vi "Do Non-Critical Stuff.vi"() -> ()   [LabVIEW 2017]
panel:
  out "Torque Chart":dbl(graph)
  out "Uncertainty Contributions":dbl[](array[numeric])
  out "Discharge Pressure Random Uncertainty":dbl
  out "Suction Pressure Random Uncertainty":dbl
  out "Suction Temperature Random Uncertainty":dbl
  out "size(s)":i32
  out "varclusterarray":T1(array[cluster])
  in  "units":enum16{"SI", "IP"}(ring)
  out "Hevap,inlet":string
  out "Psat(130F)":string
  out "Density":string
  out "Psat(45F)":string
  out "x > y?":bool
  out "x .and. y?":bool
  out "queue out":refnum<queue>
  out "DT Subcool":dbl
  out "DT Superheat":dbl
  out "Volumetric Efficiency":dbl
  out "Capacity":dbl
  out "Isentropic Efficiency":dbl
  in  "Tab Control":enum32{"Test Information", "Test Data"}(tab)
  in  "Test Matrix File":path=path "C:/Users/betsrgadmin/Desktop/80_Labview/80_Ton_Labview/test_matrix_labview_40ton_1234ze.csv"
  in  "Systematic Uncertainty of Pdis":dbl=0.375
  in  "Systematic Uncertainty of Psuc":dbl=0.1
  in  "Systematic Uncertainty of Tsuc":dbl=0.2
  in  "Build Sheet Directory":path=path "C:/Users/betsrgadmin/Desktop/80_Labview/80_Ton_Labview/Build_Sheets"
  in  "Data Root Directory":path=path "C:/Users/betsrgadmin/Desktop/80_Labview/80_Ton_Labview/Test_Data"
  in  "Debug?":bool
  in  "Fluid":u16(ring)=220 items=["AIR.MIX", "AMARILLO.MIX", "EKOFISK.MIX", "GLFCOAST.MIX", "HIGHCO2.MIX", "HIGHN2.MIX", "NGSAMPLE.MIX", "R401A.MIX", "R401B.MIX", "R401C.MIX", "R402A.MIX", "R402B.MIX", "R403A.MIX", "R403B.MIX", "R405A.MIX", "R406A.MIX", "R407A.MIX", "R407B.MIX", "R407C.MIX", "R407D.MIX", "R407E.MIX", "R408A.MIX", "R409A.MIX", "R409B.MIX", "R410A.PPF", "R410B.MIX", "R411A.MIX", "R411B.MIX", "R412A.MIX", "R413A.MIX", "R414B.MIX", "R415A.MIX", "R415B.MIX", "R416A.MIX", "R417A.MIX", "R417B.MIX", "R417C.MIX", "R418A.MIX", "R419A.MIX", "R419B.MIX", "R420A.MIX", "R421A.MIX", "R421B.MIX", "R422A.MIX", "R422B.MIX", "R422C.MIX", "R422D.MIX", "R423A.MIX", "R424A.MIX", "R425A.MIX", "R426A.MIX", "R427A.MIX", "R428A.MIX", "R429A.MIX", "R430A.MIX", "R431A.MIX", "R432A.MIX", "R433A.MIX", "R433B.MIX", "R433C.MIX", "R434A.MIX", "R435A.MIX", "R436A.MIX", "R436B.MIX", "R437A.MIX", "R438A.MIX", "R439A.MIX", "R440A.MIX", "R441A.MIX", "R442A.MIX", "R443A.MIX", "R444A.MIX", "R444B.MIX", "R445A.MIX", "R446A.MIX", "R447A.MIX", "R448A.MIX", "R449A.MIX", "R449B.MIX", "R450A.MIX", "R451A.MIX", "R451B.MIX", "R452A.MIX", "R452B.MIX", "R452C.MIX", "R453A.MIX", "R454A.MIX", "R454B.MIX", "R454C.MIX", "R455A.MIX", "R456A.MIX", "R457A.MIX", "R459A.MIX", "R459B.MIX", "R460A.MIX", "R460B.MIX", "R500.MIX", "R501.MIX", "R502.MIX", "R503.MIX", "R504.MIX", "R507A.MIX", "R508A.MIX", "R508B.MIX", "R509A.MIX", "R510A.MIX", "R511A.MIX", "R512A.MIX", "R513A.MIX", "R513B.MIX", "R515A.MIX", "ammonia.fld", "butane.fld", "ethane.fld", "propane.fld", "R11.fld", "R113.fld", "R114.fld", "R115.fld", "R116.fld", "R12.fld", "R123.fld", "R124.fld", "R125.fld", "R13.fld", "R134a.fld", "R14.fld", "R141b.fld", "R142b.fld", "R143a.fld", "R152a.fld", "R161.fld", "R21.fld", "R218.fld", "R22.fld", "R227ea.fld", "R23.fld", "R236ea.fld", "R236fa.fld", "R245ca.fld", "R245fa.fld", "R32.fld", "R41.fld", "R1216.fld", "RC318.fld", "water.fld", "1butene.fld", "acetone.fld", "argon.fld", "benzene.fld", "c1cc6.fld", "c2butene.fld", "c3cc6.fld", "c4f10.fld", "c5f12.fld", "c11.fld", "c12.fld", "cf3i.fld", "CO.fld", "CO2.fld", "COS.fld", "cyclohex.fld", "cyclopen.fld", "cyclopro.fld", "D2.fld", "D2O.fld", "D4.fld", "D5.fld", "D6.fld", "decane.fld", "dee.fld", "dmc.fld", "dme.fld", "ebenzene.fld", "ethanol.fld", "ethylene.fld", "flourine.fld", "H2S.fld", "HCl.fld", "helium.fld", "heptane.fld", "hexane.fld", "hydrogen.fld", "ibutene.fld", "ihexane.fld", "ioctane.fld", "ipentane.fld", "isobutan.fld", "krypton.fld", "MD2M.fld", "MD3M.fld", "MD4M.fld", "MDM.fld", "methane.fld", "methanol.fld", "mlinolea.fld", "mlinolen.fld", "MM.fld", "moleate.fld", "mpalmita.fld", "mstearat.fld", "mxylene.fld", "N2O.fld", "neon.fld", "neopentn.fld", "NF3.fld", "nitrogen.fld", "nonane.fld", "novec649.fld", "octane.fld", "orthohyd.fld", "oxygen.fld", "parahyd.fld", "pentane.fld", "propylen.fld", "propyne.fld", "pxylene.fld", "R365MFC.fld", "R1233zd.fld", "R1234yf.fld", "R1234ze.fld", "RE143a.fld", "RE245cb2.fld", "RE245fa2.fld", "RE347mcc.fld", "sf6.fld", "SO2.fld", "T2butene.fld", "xenon.fld"]
  out "Number in Queue":i32
  in  "Save Data":bool
  in  "Override Build\nFile Write":bool=TRUE
  in  "Purpose of Test (NO COMMAS)":string
  in  "Tester":string(combo)="J Singleton"
  in  "Test Comments (NO COMMAS)":string
  in  "Build Number":string="40TonSpool_ze"
  in  "Test Request\n    Number":string="1"
  out "Raw Data Directory Path":path
  out "Raw Data File Path":path
  in  "Points to Aquire":i32=1000
  in  "Compressor Displacement Volume (m^3)":dbl=0.002143428
  in  "Nominal Rotational Speed Hz":dbl=60.0
  out "Nominal Capacity kW":dbl
  in  "Units":string(combo)="IP"
  in  "# Motor Poles":dbl=4.0
  in  "Dump Queue":bool
  in  "Test Number in Matrix you want\n(Use this if manually changing to new setpoint. Otherwise, SP will change automatically when saved.)":i32=1
  out "Number in matrix being tested":i32
  out "Total Suction Temperature Uncertainty":dbl
  out "Total Suction Pressure Uncertainty":dbl
  out "Total Discharge Pressure Uncertainty":dbl
  out "Psuc Random Contribution to Total":dbl
  out "Tsuc Random Contribution to Total":dbl
  out "Pdis Random Contribution to Total":dbl
  in  "Collect Transient":bool
  in  "percentage of random uncertainty allowed":dbl=10.0 format="%#_13g"
  in  "Economizer used?":bool
  out "?":cluster{dbl, string, string}[](array[cluster])
  out "?":cluster{dbl, string, string}[](array[cluster])
  in  "?":T2(tab)
  in  "?":T3(tab)
  out "Primary Pressure Plot":dbl[][](graph)
  out "Secondary Pressure Plot":dbl[][](graph)
  out "Primary Pressure Plot 2":dbl[][](graph)
  in  "?":T4(tab)
  out "Primary Temperature Plot":dbl[][](graph)
  out "Secondary Temperature Plot":dbl[][](graph)
  out "Primary Temperature Plot 2":dbl[][](graph)
  out "Oil Mass Flow Plot":dbl[][](graph)
  out "Mass Flow Plot":dbl[][](graph)
  out "DTsup/DTsub Plot":dbl[][](graph)
  out "Efficiency Plot":dbl[][](graph)
  out "?":dbl[][](graph)
  out "Random uncertainties":dbl[][](graph)
  out "?":cluster{dbl, string, string}[](array[cluster]) {"?" format="%#_5g"}
  out "?":cluster{dbl, string, string}[](array[cluster]) {"?" format="%#_3g"}
  out "?":cluster{dbl, string, string}[](array[cluster]) {"?" format="%#_3g"}
  out "?":cluster{dbl, string, string}[](array[cluster]) {"?" format="%#_4g"}
  in  "stop":bool
  out "?":cluster{dbl, string, string}[](array[cluster])
  out "?":cluster{dbl, string, string}[](array[cluster])
  # "Seth was present here."
  # "Test Information"
  # "Compressor Information"
  # "Data Collection Information"
  # "Code will automatically save the test \ncondtion when the uncertainty is \nminimized. The condition can be saved \nmanually by pressing \"Save Data\""
  # "The code will not begin queuing data until the pressures\nare within +/- 1% and the temperature is within +/-\n1 F of the setpoint (ASHRAE  2010 compressor testing \nstandard). If a different threshold is desired, or a \ntransient condition is being tested, press \"Collect Transient\" to begin queuing data."
  # "Measurement Plots"
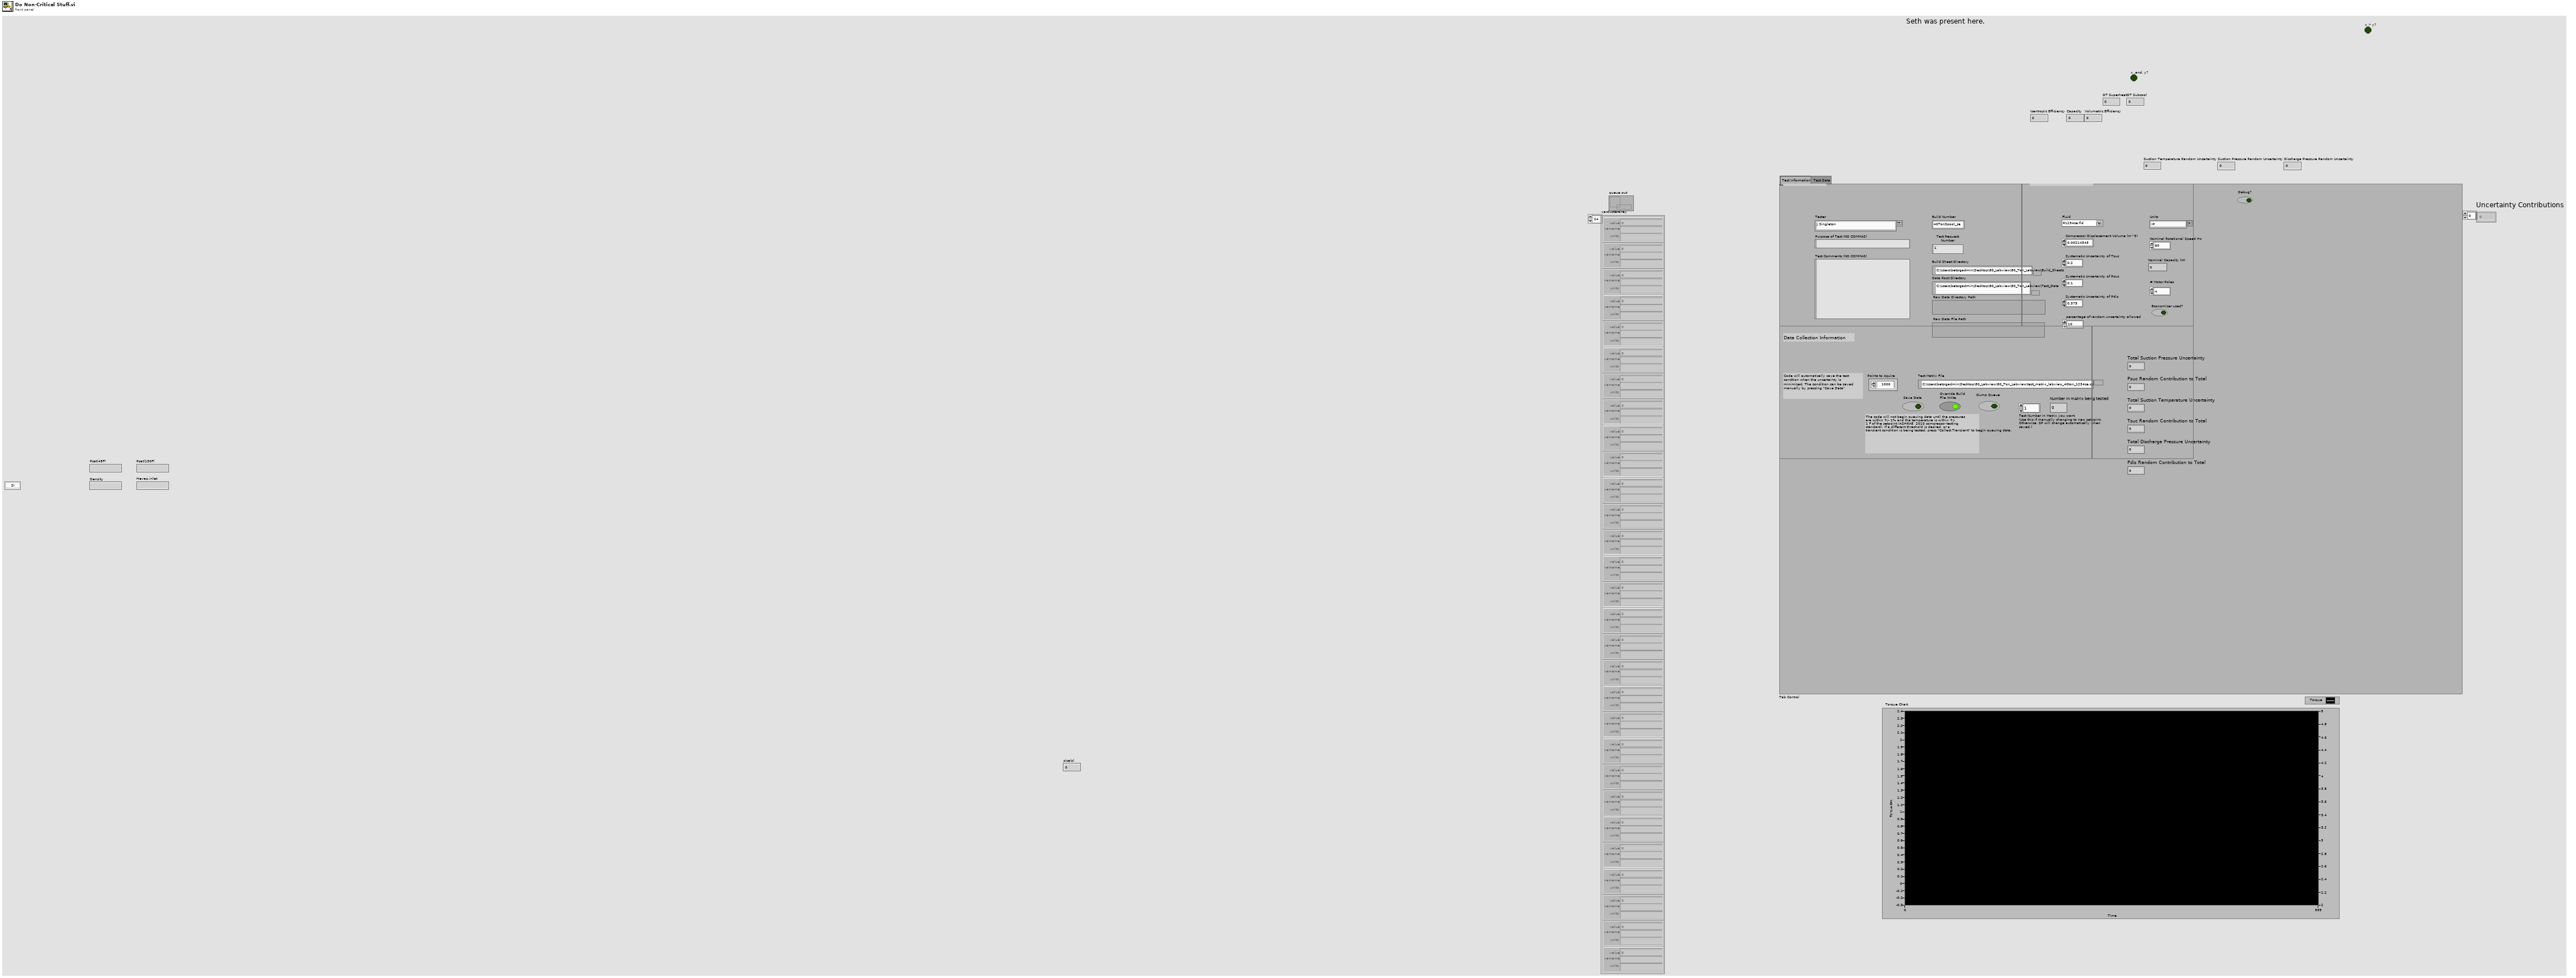
[diagram p1: front panel]
types:
  T1 = cluster{"value":dbl, "varname":string, "units":string}[]
  T2 = enum32{"Temperature/Pressure", "Mass Flow/Power", "Efficiency/Superheat and Subcooling", "Water Control Positions", "Uncertainty Contributions"}
  T3 = enum32{"Primary Pressure Plots", "Secondary Pressure Plots", "Pressure Queue"}
  T4 = enum32{"Primary Temperature Plots", "Secondary Temperature Plots", "Temperature Queue"}
  T5 = enum16{"0", "PS", "HS", "T", "P", "TP", "TH", "TS", "PH", "PQ", "TQ"}
  T6 = cluster{"RTDs":dbl[], "Thermocouples":dbl[], "Pressure Transducers":dbl[], "Mass Flow Meters":dbl[], "Barometer":dbl[], "Accelerometer":dbl[], "Power":dbl[], "Water Valve Position":dbl[]}
  T7 = cluster{"Build Sheet Directory":path, "File Path":path, "Directory Path":path, "Build Number":string, "Tester":string, "Purpose of Test (NO COMMAS)":string, "Test Comments (NO COMMAS) ":string, "Test Request\n    Number":string, "Data Root Directory":path}
  T8 = cluster{"queue out":refnum<queue>, "Points to Aquire":i32}
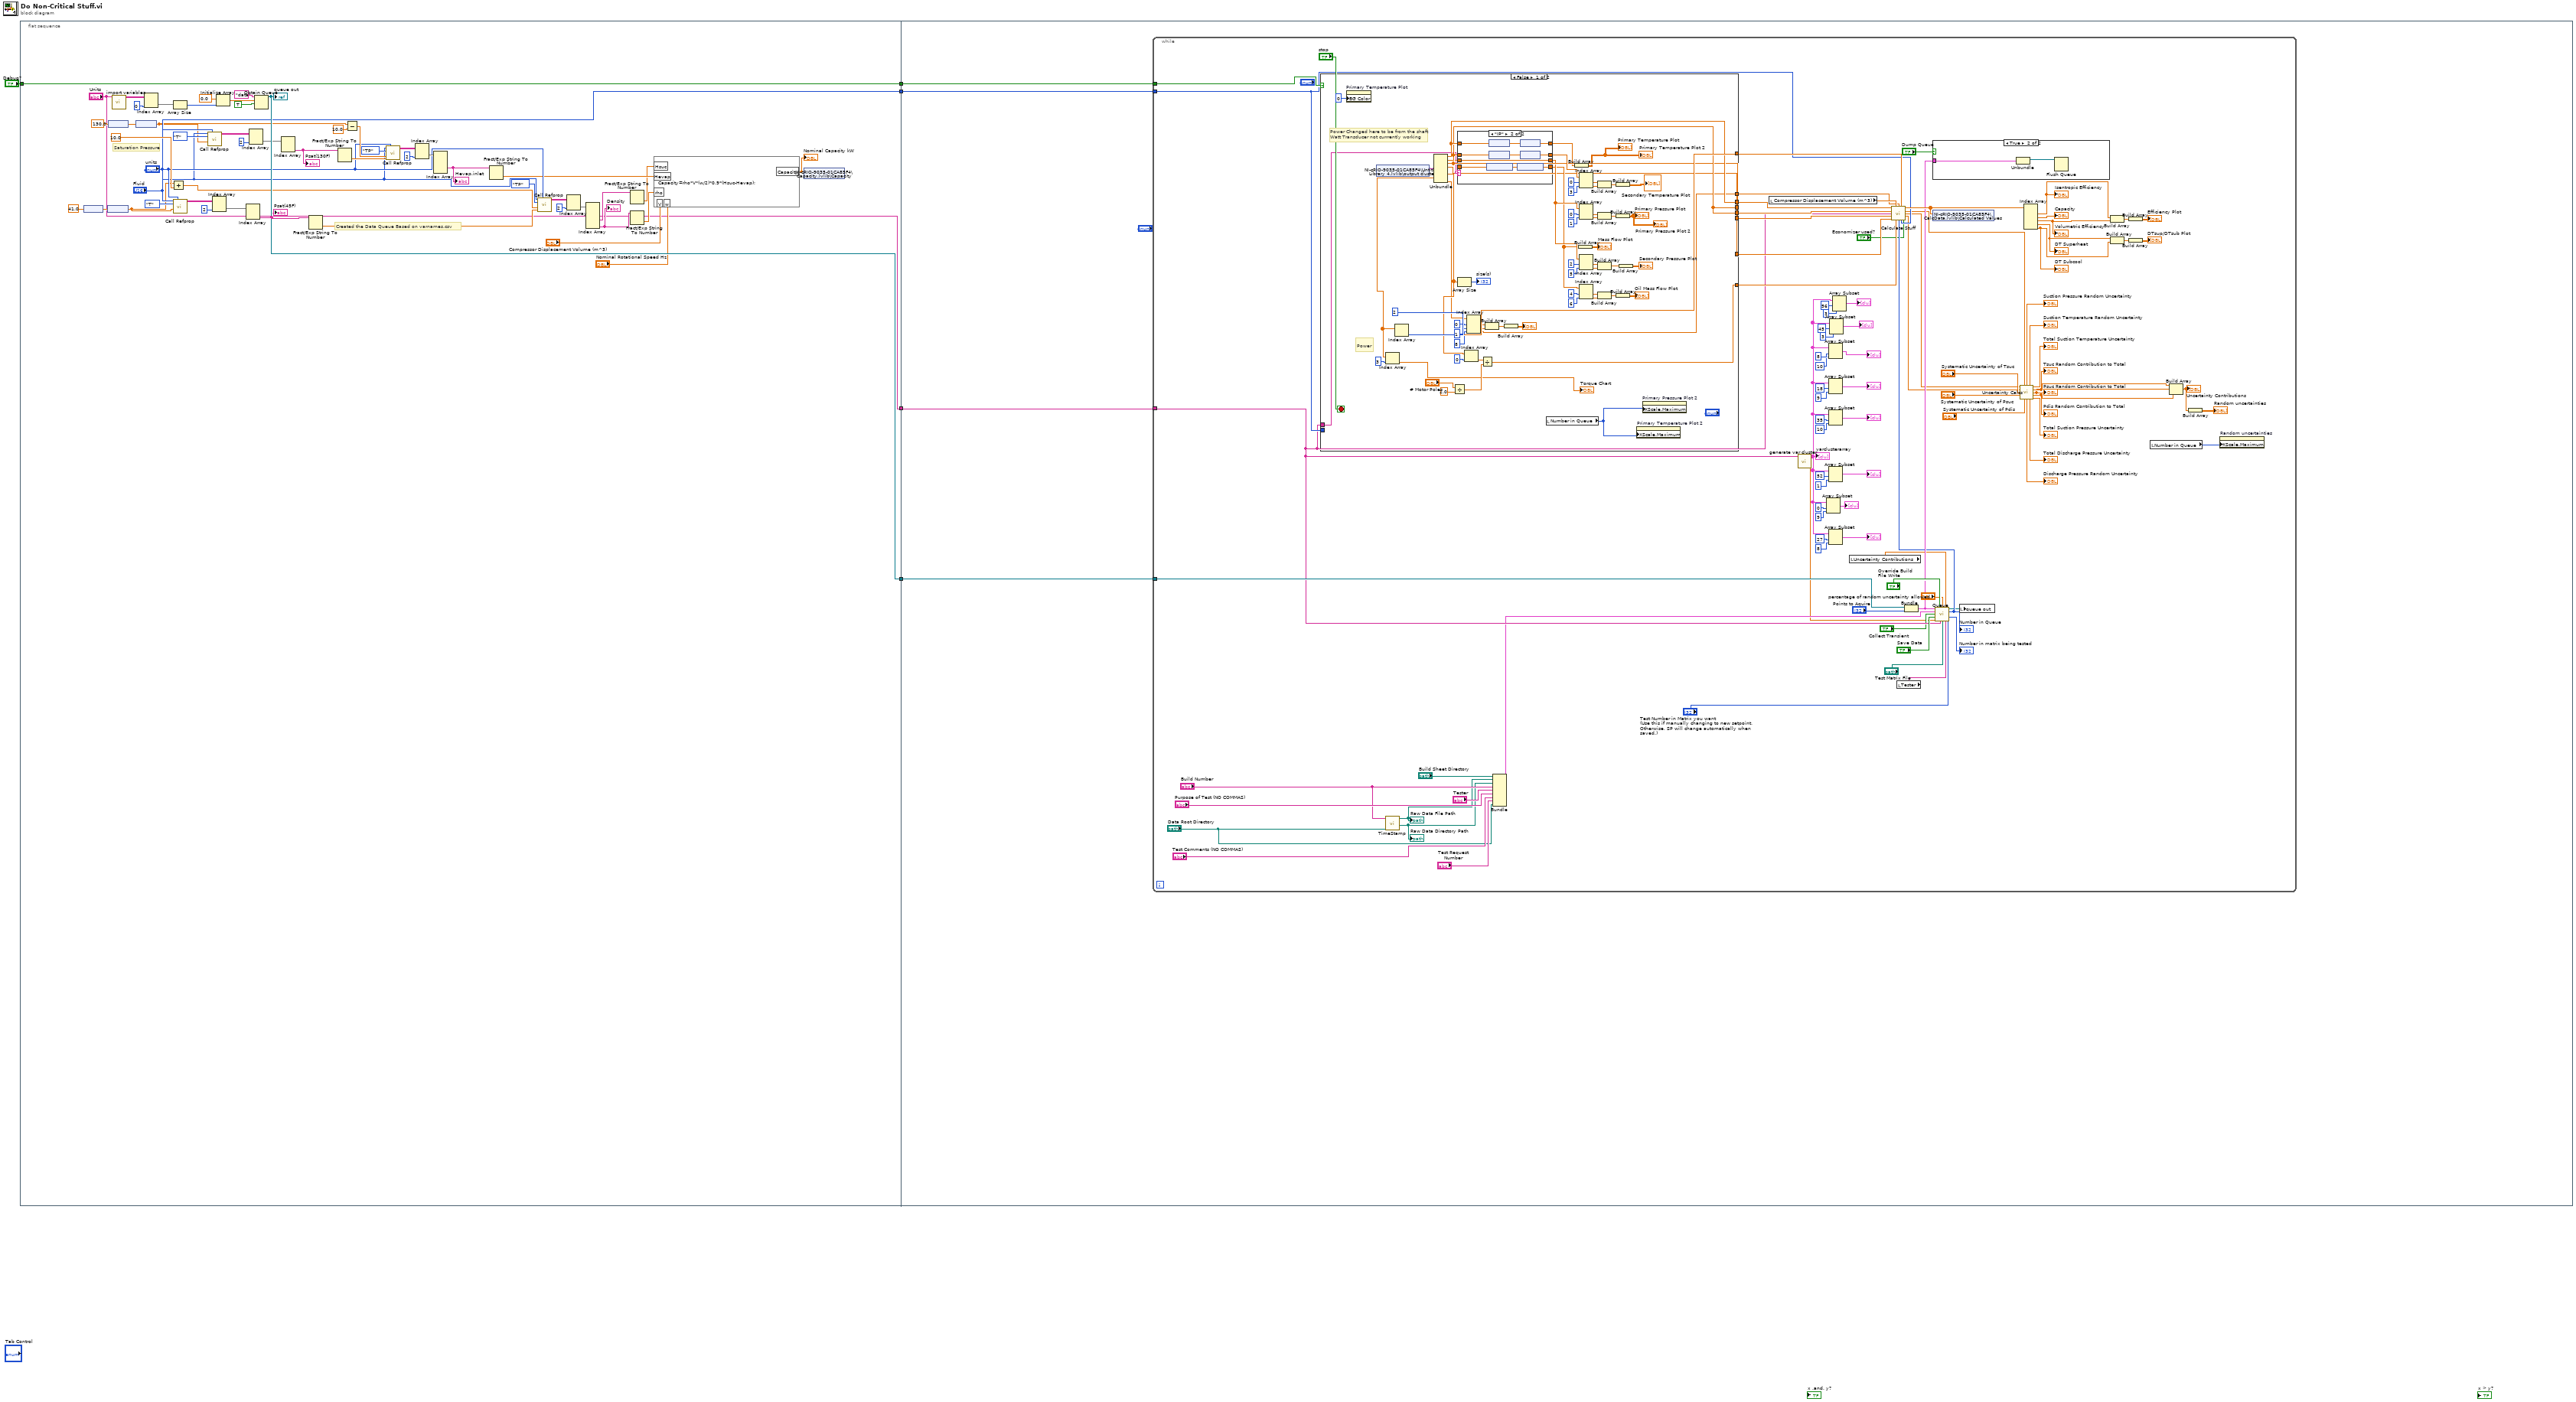
[diagram p0: block diagram]
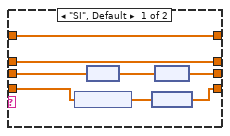
[diagram p3: hidden frame]
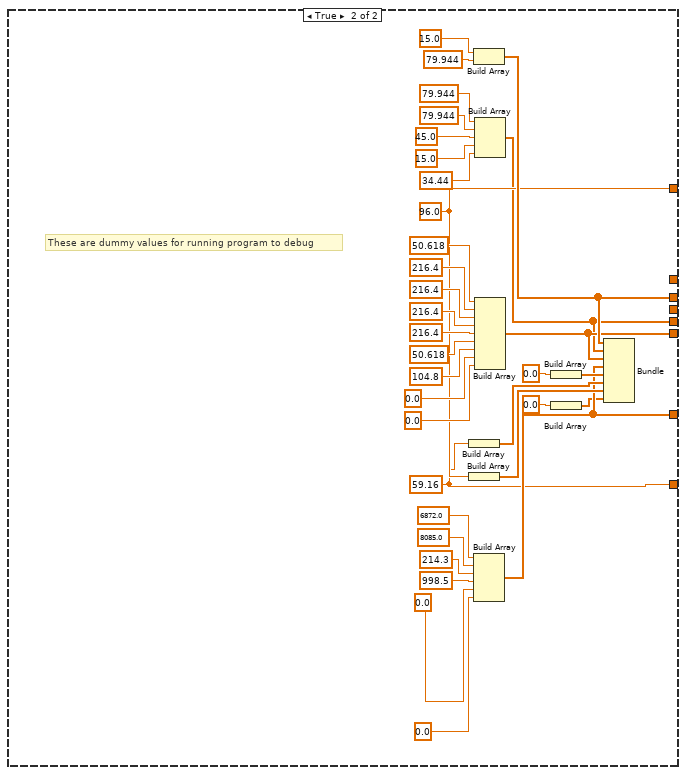
[diagram p4: hidden frame]
diagram:
  n1 = flat-sequence {
    tunnel: "Debug?" -> [w57]
    tunnel: ["Fluid"] -> w4
    tunnel: [w57] -> w3
    tunnel: [w56] -> w2
    tunnel: ["Units"] -> w1
    tunnel: w4 -> [w61]
    tunnel: w3 -> [w60]
    tunnel: w2 -> [w59]
    tunnel: w1 -> [w58]
    frame #0 {
      # "Saturation Pressure"
      # "Created the Data Queue Based on varnames.csv"
      n2 = node(41.0 ("output_1")) -> (w10:dbl[unit])
      n3 = node(w10) -> (w8:dbl)
      n4 = node(130.0 ("output_1")) -> (w13:dbl[unit])
      n5 = call "import variables.vi"("units"="Units") -> ("String Array From File"=w54:string[][])  [unwired: 9 in, 1 out]
      n6 = node(w13) -> (w11:dbl)
      n7 = Index Array(array=w54, index (col)=0 ("index (row)")) -> (element=w53:string[])  [unwired: 1 in]
      n8 = Add(x=w8, y=10.0) -> (x+y=w41:dbl)
      n9 = Array Size(array=w53) -> (size(s)=w52:i32)
      n10 = call "Call Refprop.vi"("fluid name"="Fluid", "units"="units", "InpCode"=T5."T", "output_1"=w8) -> ("data"=w46:string[][])  [unwired: 7 in, 4 out]
      n11 = call "Call Refprop.vi"("fluid name"="Fluid", "units"="units", "InpCode"=T5."T", "output_1"=w11) -> ("data"=w34:string[][])  [unwired: 7 in, 4 out]
      n12 = Index Array(array=w46, index (col)=2 ("disabled index (col)")) -> (element=w44:string[])  [unwired: 1 in]
      n13 = Initialize Array(0.0, w52) -> (w55:dbl[])
      n14 = Index Array(array=w44) -> (element #2=w37:string)  [unwired: 2 in, 1 out]
      "Psat(45F)" <- w37
      n15 = Index Array(array=w34, index (col)=2 ("disabled index (col)")) -> (element=w32:string[])  [unwired: 1 in]
      n16 = Obtain Queue(name (unnamed)="data" ("queue name"), element data type=w55, create if not found? (T)=TRUE) -> (queue out=w56:refnum<queue>)  [unwired: 2 in, 2 out]
      "queue out" <- w56
      n17 = Index Array(array=w32) -> (element #2=w31:string)  [unwired: 2 in, 1 out]
      "Psat(130F)" <- w31
      n18 = Fract/Exp String To Number(string=w37) -> (number=w36:dbl)  [unwired: 3 in, 1 out]
      n19 = Fract/Exp String To Number(string=w31) -> (number=w30:dbl)  [unwired: 3 in, 1 out]
      n20 = Subtract(x=w11, y=10.0) -> (x-y=w27:dbl)
      n21 = call "Call Refprop.vi"("fluid name"="Fluid", "units"="units", "InpCode"=T5."TP", "output_1"=w27, "output_2"=w30) -> ("data"=w26:string[][])  [unwired: 6 in, 4 out]
      n22 = Index Array(array=w26, index (col)=2 ("disabled index (col)")) -> (element=w24:string[])  [unwired: 1 in]
      n23 = Index Array(array=w24) -> (element #3=w21:string)  [unwired: 4 in, 3 out]
      "Hevap,inlet" <- w21
      n24 = Fract/Exp String To Number(string=w21) -> (number=w19:dbl)  [unwired: 3 in, 1 out]
      n25 = call "Call Refprop.vi"("fluid name"="Fluid", "units"="units", "InpCode"=T5."TP", "output_1"=w41, "output_2"=w36) -> ("data"=w40:string[][])  [unwired: 6 in, 4 out]
      n26 = Index Array(array=w40, index (col)=2 ("disabled index (col)")) -> (element=w38:string[])  [unwired: 1 in]
      n27 = Index Array(array=w38) -> (element #3=w17:string, element #5=w23:string)  [unwired: 5 in, 3 out]
      "Density" <- w23
      n28 = Fract/Exp String To Number(string=w17) -> (number=w16:dbl)  [unwired: 3 in, 1 out]
      n29 = Fract/Exp String To Number(string=w23) -> (number=w22:dbl)  [unwired: 3 in, 1 out]
      n30 = formula code="Capacity=rho*V*(w/2)*0.9*(Hsuc-Hevap);"("rho"=w22, "V"="Compressor Displacement Volume (m^3)", "w"="Nominal Rotational Speed Hz", "Hsuc"=w16, "Hevap"=w19) -> ("Capacity"=w14:dbl)
      "Nominal Capacity kW" <- w14
      n31 = shared-variable "NI-cRIO-9035-01CA85F4\\Capacity.lvlib\\Capacity"(w14) -> ()  [unwired: 1 in, 1 out]
    }
    frame #1 {
      n32 = while {
        tunnel: w61 -> [w141]
        tunnel: w60 -> [w152]
        tunnel: w59 -> [w149]
        tunnel: w58 -> [w124]
        stop <- "stop" stop-if-true
        n33 = case shown="False" w152 {
          tunnel: w141 -> [_ _]
          tunnel: [w198 w241] -> w142
          tunnel: [w156 w239] -> w144
          tunnel: [w195 w240] -> w143
          tunnel: [w214 w238] -> w146
          tunnel: [w174 w237] -> w145
          tunnel: [w197 _] -> _
          tunnel: [w197 w236] -> w127
          tunnel: w124 -> [w194 _]
          tunnel: [w165 _] -> w73
          frame False {
            # "Power"
            # "Power Changed here to be from the shaft\nWatt Transducer not currrently working"
            n34 = property on="Primary Temperature Plot" class="WFChart (strict)"("BG Color"=u32 0 ("Plot Area:Colors:BG Color")) -> ()  [unwired: 2 in, 2 out]
            n35 = shared-variable "NI-cRIO-9035-01CA85F4\\Untitled Library 4.lvlib\\output cluster"() -> (w181:T6)  [unwired: 1 in, 1 out]
            n36 = Unbundle(w181) -> ("RTDs"=w198:dbl[], "Thermocouples"=w197:dbl[], "Pressure Transducers"=w195:dbl[], "Mass Flow Meters"=w156:dbl[], "Accelerometer"=w203:dbl[], "Power"=w161:dbl[], "Water Valve Position"=w158:dbl[])  [unwired: 1 out]
            n37 = Index Array(array=w161, index=3) -> (element=→"Torque Chart":dbl)
            n38 = Index Array(array=w161, index=2) -> (element=w214:dbl)
            n39 = Divide(x="# Motor Poles", y=2.0) -> (x/y=w162:dbl)
            n40 = case shown="\"IP\"" w194 {
              tunnel: w198 -> [w223 w230]
              tunnel: [w223 w231] -> w173
              tunnel: w197 -> [w222 w228]
              tunnel: [w222 w227] -> w196
              tunnel: w195 -> [w220 w233]
              tunnel: [w219 w233] -> w185
              tunnel: w156 -> [w218 w224]
              tunnel: [w216 w225] -> w157
              frame "SI", Default {
                n41 = node(w218) -> (w217:dbl[unit][])
                n42 = node(w220) -> (w221:dbl[unit][])
                n43 = node(w217) -> (w216:dbl[])
                n44 = node(w221) -> (w219:dbl[])
              }
              frame "IP" {
                n45 = node(w224) -> (w226:dbl[unit][])
                n46 = node(w230) -> (w232:dbl[unit][])
                n47 = node(w228) -> (w229:dbl[unit][])
                n48 = node(w226) -> (w225:dbl[])
                n49 = node(w232) -> (w231:dbl[])
                n50 = node(w229) -> (w227:dbl[])
              }
            }
            n51 = Array Size(array=w203) -> (size(s)=→"size(s)":i32)
            n52 = Index Array(array=w203, index=0) -> (element=w166:dbl)
            n53 = Index Array(array=w158, index #1=0 ("index"), index #2=1 ("index"), index #3=8 ("index")) -> (element #1=w179:dbl, element #2=w178:dbl, element #3=w165:dbl)
            n54 = Divide(x=w166, y=w162) -> (x/y=w174:dbl)
            n55 = Build Array(w179, w178) -> (w180:dbl[])
            n56 = Build Array(w180) -> (→"?":dbl[][])
            n57 = local read "Number in Queue"() -> (w168:i32)
            n58 = Build Array(w173) -> (→"Primary Temperature Plot" →"Primary Temperature Plot 2":dbl[][])
            n59 = Build Array(w157) -> (→"Mass Flow Plot":dbl[][])
            n60 = Index Array(array=w196, index #1=0 ("index"), index #2=3 ("index")) -> (element #1=w206:dbl, element #2=w205:dbl)
            n61 = Index Array(array=w185, index #1=0 ("index"), index #2=1 ("index")) -> (element #1=w171:dbl, element #2=w172:dbl)
            n62 = Index Array(array=w185, index #1=2 ("index"), index #2=5 ("index")) -> (element #1=w209:dbl, element #2=w210:dbl)
            n63 = Index Array(array=w157, index #1=4 ("index"), index #2=6 ("index")) -> (element #1=w188:dbl, element #2=w187:dbl)
            n64 = Build Array(w206, w205) -> (w193:dbl[])
            n65 = Build Array(w171, w172) -> (w182:dbl[])
            n66 = Build Array(w209, w210) -> (w200:dbl[])
            n67 = Build Array(w188, w187) -> (w186:dbl[])
            n68 = Build Array(w193) -> (→"Secondary Temperature Plot":dbl[][])
            n69 = Build Array(w182) -> (→"Primary Pressure Plot" →"Primary Pressure Plot 2":dbl[][])
            n70 = Build Array(w186) -> (→"Oil Mass Flow Plot":dbl[][])
            n71 = Build Array(w200) -> (→"Secondary Pressure Plot":dbl[][])
            n72 = property on="Primary Temperature Plot 2" class="WFChart (strict)"("XScale.Maximum"=w168) -> ()  [unwired: 2 in, 2 out]
            n73 = property on="Primary Pressure Plot 2" class="WFChart (strict)"("XScale.Maximum"=w168) -> ()  [unwired: 2 in, 2 out]
          }
          frame True {
            w238 = 96.0 ("element")
            w237 = 59.16 ("element")
            # "These are dummy values for running program to debug"
            n74 = Build Array(w237) -> (w243:dbl[])
            n75 = Build Array(w238) -> (w242:dbl[])
            n76 = Build Array(15.0 ("element"), 79.944 ("element")) -> (w241:dbl[])
            n77 = Build Array(6872.0 ("element"), 8085.0 ("element"), 214.3 ("element"), 998.5 ("element"), 0.0 ("element"), 0.0 ("element")) -> (w239:dbl[])
            n78 = Build Array(79.944 ("element"), 79.944 ("element"), 45.0 ("element"), 15.0 ("element"), 34.44 ("element")) -> (w236:dbl[])
            n79 = Build Array(50.618 ("element"), 216.4 ("element"), 216.4 ("element"), 216.4 ("element"), 216.4 ("element"), 50.618 ("element"), 104.8 ("element"), 0.0 ("element"), 0.0 ("element")) -> (w240:dbl[])
            n80 = Build Array(0.0 ("element")) -> (w244:dbl[])
            n81 = Build Array(0.0 ("element")) -> (w234:dbl[])
            n82 = Bundle(w241, w236, w240, w239, w244, w243, w242, w234) -> ()  [unwired: 1 in, 1 out]
          }
        }
        n83 = call "TimeStamp.vi"("Root Path"="Data Root Directory", "Build Name"="Build Number") -> ("Directory Path"=w77:path, "File Path"=w78:path)  [unwired: 7 in, 1 out]
        "Raw Data Directory Path" <- w77
        "Raw Data File Path" <- w78
        n84 = Bundle("Build Sheet Directory"="Build Sheet Directory", "File Path"=w78, "Directory Path"=w77, "Build Number"="Build Number", "Tester"="Tester", "Purpose of Test (NO COMMAS)"="Purpose of Test (NO COMMAS)", "Test Comments (NO COMMAS)"="Test Comments (NO COMMAS)", "Test Request\n    Number"="Test Request\n    Number", "Data Root Directory"="Data Root Directory") -> (w74:T7)  [unwired: 1 in]
        n85 = local read "Compressor Displacement Volume (m^3)"() -> (w140:dbl)
        n86 = call "generate var cluster.vi"("Units"=w124) -> ("numarray"=w65:dbl[], "varclusterarray"=w67:T1)  [unwired: 7 in, 2 out]
        "varclusterarray" <- w67
        n87 = Array Subset(array=w67, index=0, length=9) -> (→"?":T1)
        n88 = Array Subset(array=w67, index=8, length=10) -> (→"?":T1)
        n89 = Array Subset(array=w67, index=18, length=9) -> (→"?":T1)
        n90 = Array Subset(array=w67, index=35, length=10) -> (→"?":T1)
        n91 = Array Subset(array=w67, index=52, length=1) -> (→"?":T1)
        n92 = Array Subset(array=w67, index=27, length=8) -> (→"?":T1)
        n93 = Array Subset(array=w67, index=45, length=3) -> (→"?":T1)
        n94 = Array Subset(array=w67, index=56, length=3) -> (→"?":T1)
        n95 = local read "Uncertainty Contributions"() -> (w93:dbl[])
        n96 = local read "Tester"() -> (w90:string)
        n97 = Bundle("queue out"=w149, "Points to Aquire"="Points to Aquire") -> (w110:T8)  [unwired: 1 in]
        n98 = case shown="True" "Dump Queue" {
          tunnel: w110 -> [_ w155]
          frame False {
          }
          frame True {
            n99 = Unbundle(w155) -> ("queue out"=w154:refnum<queue>)  [unwired: 1 out]
            n100 = Flush Queue(queue=w154) -> ()  [unwired: 1 in, 3 out]
          }
        }
        n101 = call "Queue.vi"("Cluster"=w110, "Override Build\nFile Write"="Override Build\nFile Write", "percentage of random uncertainty allowed"="percentage of random uncertainty allowed", "Uncertainty Contributions"=w93, "Saving Cluster"=w74, "Collect Transient"="Collect Transient", "Save Data"="Save Data", "Data In"=w65, "units"=w124, "file path (dialog if empty)"="Test Matrix File", "Tester"=w90, "Loop Iter"="Test Number in Matrix you want\n(Use this if manually changing to new setpoint. Otherwise, SP will change automatically when saved.)") -> ("queue out"=w63:refnum<queue>, "Number in Queue"=w109:i32, "Numeric"=→"Number in matrix being tested":i32)  [unwired: 1 in]
        "Number in Queue" <- w109
        n102 = call "Calculate Stuff.vi"("RTD in"=w142, "Compressor Displacement Volume"=w140, "VFD power"=w73, "Power (kW)"=w146, "TC in"=w127, "Units"=w124, "P in"=w143, "mdot in"=w144, "Compressor Rotational Speed"=w145, "Number in Queue"=w109, "fluid name"=w141, "Economizer used?"="Economizer used?") -> ("Calculated Values"=w148:dbl[], "Suction Temperature Random Uncertainty"=w105:dbl, "Suction Pressure Random Uncertainty"=w104:dbl, "Discharge Pressure Random Uncertainty"=w103:dbl)
        n103 = shared-variable "NI-cRIO-9035-01CA85F4\\CalcData.lvlib\\Calculated Values"(w148) -> ()  [unwired: 1 in, 1 out]
        n104 = local write "queue out"(w63) -> ()
        n105 = call "Uncertainty Calcs.vi"("Suction Pressure Random Uncertainty in"=w104, "Suction Temperature Random Uncertainty in"=w105, "Discharge Pressure Random Uncertainty in"=w103, "Systematic Uncertainty of Tsuc"="Systematic Uncertainty of Tsuc", "Systematic Uncertainty of Psuc"="Systematic Uncertainty of Psuc", "Systematic Uncertainty of Pdis"="Systematic Uncertainty of Pdis") -> ("Suction Pressure Random Uncertainty out"=→"Suction Pressure Random Uncertainty":dbl, "Suction Temperature Random Uncertainty out"=→"Suction Temperature Random Uncertainty":dbl, "Total Suction Temperature Uncertainty"=→"Total Suction Temperature Uncertainty":dbl, "Tsuc Random Contribution to Total"=w96:dbl, "Psuc Random Contribution to Total"=w95:dbl, "Pdis Random Contribution to Total"=w94:dbl, "Discharge Pressure Random Uncertainty out"=→"Discharge Pressure Random Uncertainty":dbl, "Total Discharge Pressure Uncertainty"=→"Total Discharge Pressure Uncertainty":dbl, "Total Suction Pressure Uncertainty"=→"Total Suction Pressure Uncertainty":dbl)  [unwired: 1 in]
        "Tsuc Random Contribution to Total" <- w96
        "Psuc Random Contribution to Total" <- w95
        "Pdis Random Contribution to Total" <- w94
        n106 = Index Array(array=w148) -> (element #1=w126:dbl, element #2=→"Capacity":dbl, element #3=w125:dbl, element #4=w121:dbl, element #5=w120:dbl)  [unwired: 5 in]
        "Volumetric Efficiency" <- w125
        "DT Superheat" <- w121
        "DT Subcool" <- w120
        "Isentropic Efficiency" <- w126
        n107 = Build Array(w126, w125) -> (w123:dbl[])
        n108 = Build Array(w121, w120) -> (w119:dbl[])
        n109 = Build Array(w123) -> (→"Efficiency Plot":dbl[][])
        n110 = Build Array(w119) -> (→"DTsup/DTsub Plot":dbl[][])
        n111 = local read "Number in Queue"() -> (w89:i32)
        n112 = Build Array(w96, w95, w94) -> (w92:dbl[])
        "Uncertainty Contributions" <- w92
        n113 = Build Array(w92) -> (→"Random uncertainties":dbl[][])
        n114 = property on="Random uncertainties" class="WFChart (strict)"("XScale.Maximum"=w89) -> ()  [unwired: 2 in, 2 out]
      }
    }
  }
